vi "Numeric to Variable Cluster.vi"(9 "Numeric":i32, 10 "Variable Name":string) -> (2 "Variable Cluster":T1)   [LabVIEW 2009]
panel:
  out "variant":variant
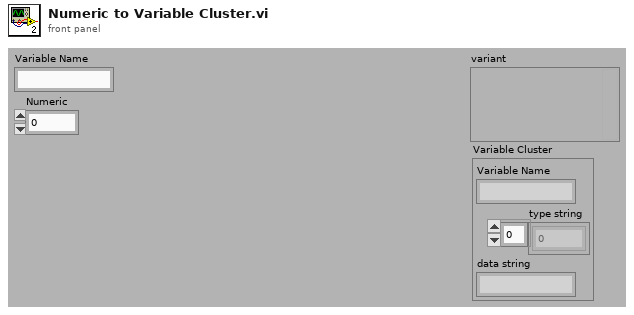
[diagram p1: front panel]
types:
  T1 = cluster{"Variable Name":string, "type string":i16[], "data string":string}
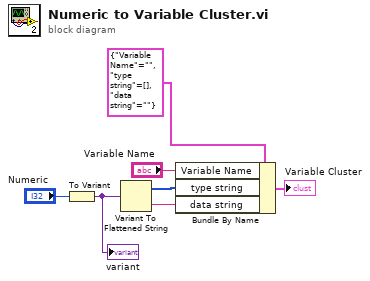
[diagram p0: block diagram]
diagram:
  n1 = To Variant(anything="Numeric") -> (Variant=w6:variant)
  "variant" <- w6
  n2 = Variant To Flattened String(Variant=w6) -> (data string=w2:string, 1:w3:i16[])
  n3 = Bundle By Name(cluster=T1 {"Variable Name"="", "type string"=[], "data string"=""} ("Variable Data"), "Variable Name"="Variable Name", "type string"=w3, "data string"=w2) -> (→"Variable Cluster":T1)
